vi "Launch Actors.vi"(8 "error in (no error)":errorcluster, 10 "Selcted Actors":string[](array[string]), 11 "CS++StartActor in":refnum<class "CS++StartActor.lvclass">) -> (0 "error out":errorcluster, 3 "CS++StartActor out":refnum<class "CS++StartActor.lvclass">)   [LabVIEW 2013, in "CS++StartActor.lvlib" / "CS++StartActor.lvclass"]
doc: "Launch Start Actors."
uses:
  CS++StartActor.lvclass
  CS++BaseActor/CS++BaseActor.lvclass/CS++BaseActor.ctl
  <vilib>/ActorFramework/Actor/Actor.lvclass/Actor.ctl
  <vilib>/ActorFramework/Message Enqueuer/Message Enqueuer.lvclass/Message Enqueuer.ctl
  CS++StartActor.lvclass/CS++StartActor.ctl
  CS++BaseActor Messages/Open Actor Core FP Msg/Open Actor Core FP Msg.lvclass/Open Actor Core FP Msg.ctl
  <vilib>/ActorFramework/Message Enqueuer/Init from Existing Queue.vi
  <vilib>/ActorFramework/Message Enqueuer/Enqueue.vi
  <vilib>/ActorFramework/Message Priority Queue/Priority Enqueue.vi
  <vilib>/ActorFramework/Message Enqueuer/Message Enqueuer.lvclass
  CS++BaseActor Messages/Open Actor Core FP Msg/Open Actor Core FP Msg.lvclass
  <vilib>/ActorFramework/Actor/Actor.lvclass
  Classes/CS++BaseClasses/Factory/CS++Factory.lvclass
  CS++BaseActor/CS++BaseActor.lvclass
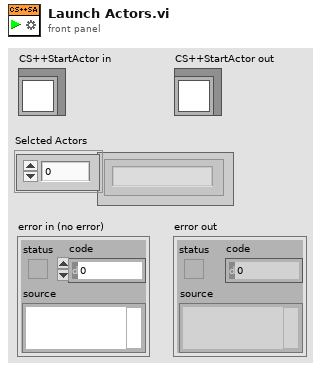
[diagram p1: front panel]
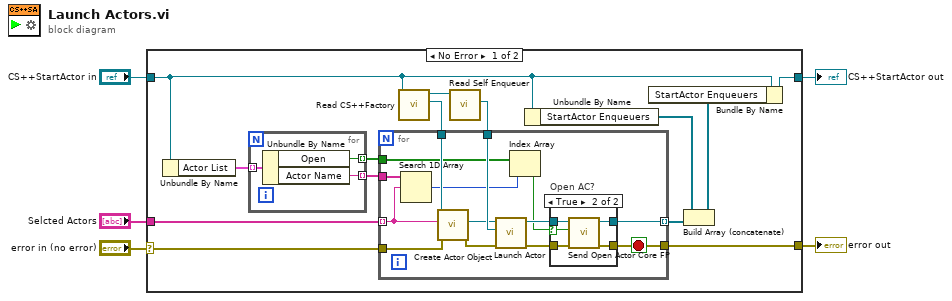
[diagram p0: block diagram]
diagram:
  n1 = case shown="No Error" "error in (no error)" {
    selector: "error in (no error)" -> [w18 w45]
    tunnel: [w11 w45] -> w4
    tunnel: [w14 w44] -> w2
    tunnel: "CS++StartActor in" -> [w10 w44]
    tunnel: "Selcted Actors" -> [w15 _]
    frame No Error {
      n2 = Unbundle By Name(w10) -> ("Actor List"=w8:cluster{"Actor Name":string, "Open":bool}[])
      n3 = for {
        tunnel: w8 -> [w22] mode=indexing
        tunnel: [w21] -> w6 mode=indexing
        tunnel: [w20] -> w7 mode=indexing
        n4 = Unbundle By Name(w22) -> ("Open"=w21:bool, "Actor Name"=w20:string)
      }
      n5 = call "Read CS++Factory.vi"("CS++BaseActor in"=w10) -> ("CS++Factory"=w17:refnum<class "CS++Factory.lvclass">, "CS++BaseActor out"=w9:refnum<class "CS++StartActor.lvclass">)  [unwired: 8 in, 1 out]
      n6 = call <vilib>:"Read Self Enqueuer.vi"("Actor"=w9) -> ("Self Enqueuer"=w19:refnum<class "Message Enqueuer.lvclass">)  [unwired: 10 in]
      n7 = for {
        tunnel: w19 -> [w36]
        tunnel: w15 -> [w27] mode=indexing
        tunnel: w17 -> [w34]
        tunnel: w18 -> [w33]
        tunnel: [w30] -> w11
        tunnel: [w28] -> w16 mode=indexing
        tunnel: w7 -> [w26]
        tunnel: w6 -> [w25]
        stop <- w30 stop-if-true
        n8 = Search 1D Array(1D array=w26, element=w27) -> (index of element=w24:i32)  [unwired: 1 in]
        n9 = call "Create Actor Object.vi"("error in (no error)"=w33, "Object Name"=w27, "CS++Factory in"=w34) -> ("error out"=w32:errorcluster, "C++BaseActor"=w35:refnum<class "CS++BaseActor.lvclass">)  [unwired: 5 in, 2 out]
        n10 = call <vilib>:"Launch Actor.vi"("error in (no error)"=w32, "Actor-to-Caller Enqueuer"=w36, "Actor"=w35) -> ("error out"=w31:errorcluster, "Caller-To-Actor Enqueuer"=w29:refnum<class "Message Enqueuer.lvclass">)  [unwired: 7 in]
        n11 = Index Array(array=w25, index=w24) -> (element=w23:bool)
        n12 = case "Open AC?" shown="True" w23 {
          selector: w23 -> [_ w39]
          tunnel: w31 -> [w37 w43]
          tunnel: [w37 w42] -> w30
          tunnel: w29 -> [w38 w41]
          tunnel: [w38 w40] -> w28
          frame False {
          }
          frame True {
            n13 = call "Send Open Actor Core FP.vi"("error in (no error)"=w43, "Open FP (F)"=w39, "Message Enqueuer"=w41) -> ("error out"=w42:errorcluster, "Message Enqueuer out"=w40:refnum<class "Message Enqueuer.lvclass">)  [unwired: 7 in]
          }
        }
      }
      n14 = Unbundle By Name(w10) -> ("StartActor Enqueuers"=w12:refnum<class "Message Enqueuer.lvclass">[])
      n15 = Build Array (concatenate)(w12, w16) -> (w13:refnum<class "Message Enqueuer.lvclass">[])
      n16 = Bundle By Name(cluster=w10, "StartActor Enqueuers"=w13) -> (w14:refnum<class "CS++StartActor.lvclass">)
    }
    frame Error {
    }
  }
  "error out" <- w4
  "CS++StartActor out" <- w2
